vi "Misc整体图.vi"() -> ()   [LabVIEW 2014]
panel:
  in  "Access":bool
  in  "Weather":bool
  in  "Toys":bool
  in  "Tip":bool
  in  "Bookcase":bool
  in  "Agent":bool
  in  "Acroread":bool
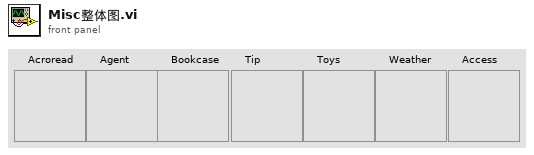
[diagram p1: front panel]
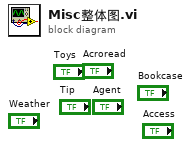
[diagram p0: block diagram]
diagram:
